vi "Dark Current Test_First_Half_Sub_VI.vi"(0 "VISA Refnum in":refnum<visa-resource-name>, 1 "Channel #":i32, 2 "dt (s)":i32, 3 "Barcodes in":string[](array[string]), 8 "N":i32) -> (10 "Actual Voltage Level (V)":dbl format="%#_13g", 12 "OVV?":bool=TRUE, 14 "Power Supply Trip":bool, 16 "OVC?":bool=TRUE, 17 "Boolean 2":bool, 18 "Actual Current Limit (nA)":dbl format="%#_13g", 19 "BoardHandle out 2":T1, 20 "VISA Refnum out":refnum<visa-resource-name>, 21 "Time Left (s)":dbl, 22 "Manual Measurments \nNeeded":bool, 23 "Barcodes out":string[](array[string]), 24 "Boolean":bool, 25 "Channel # 3":i32, 26 "Array":dbl[](array[numeric]), 27 "error out":errorcluster)   [LabVIEW 2018]
uses:
  Program Files (x86)/National Instruments/LabVIEW 2020/instr.lib/CAEN PSM/CAEN PSM.lvlib
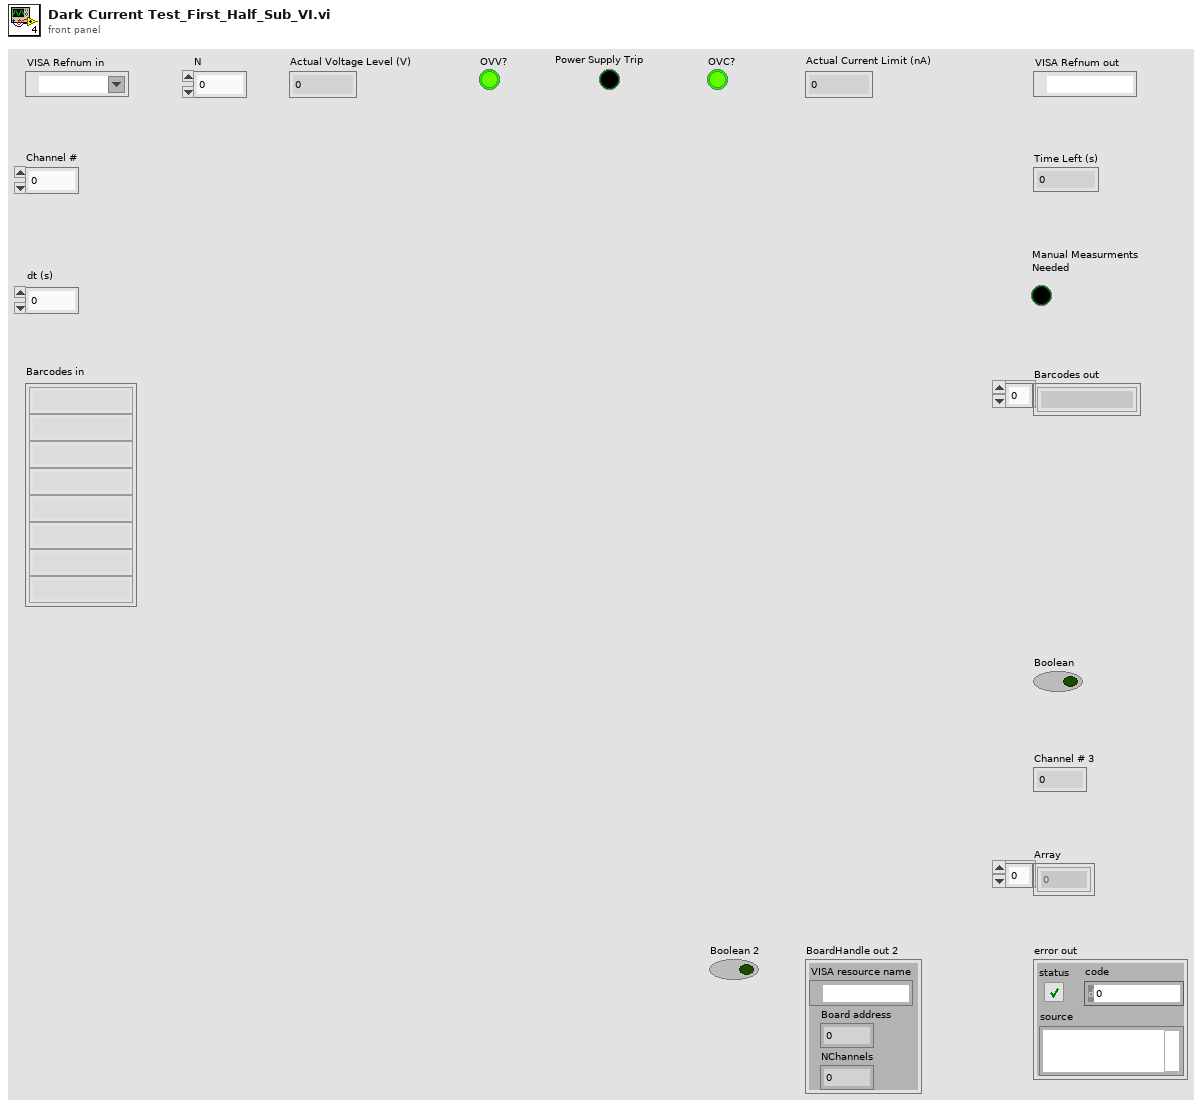
[diagram p1: front panel]
types:
  T1 = cluster{"VISA resource name":refnum<visa-resource-name>, "Board address":u8, "NChannels":u8}
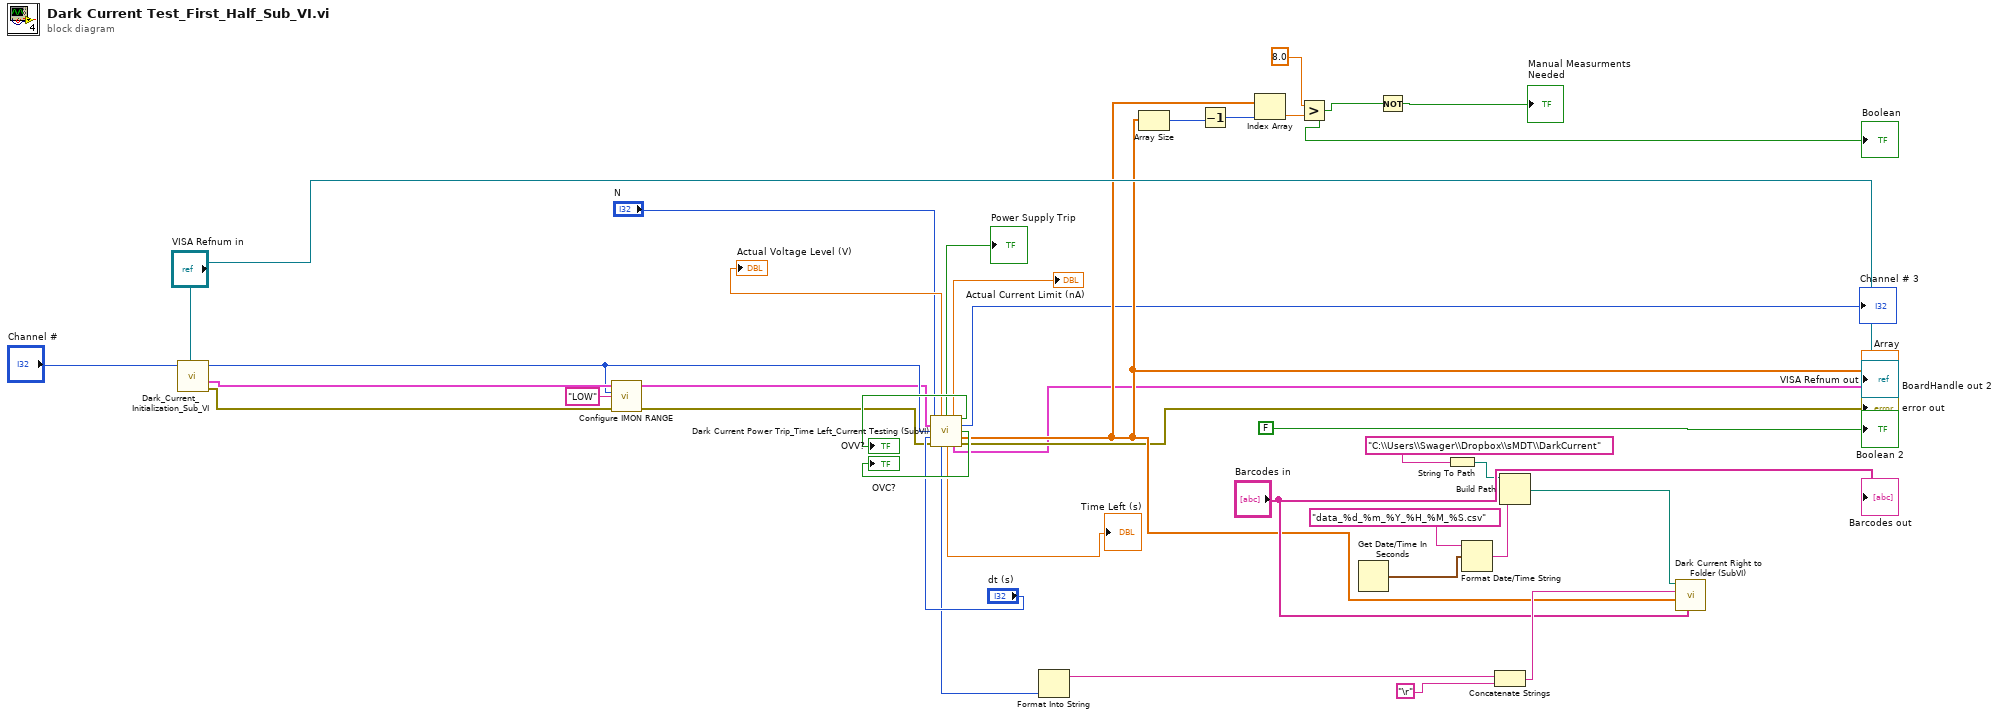
[diagram p0: block diagram]
diagram:
  n1 = call "Dark_Current_Initialization_Sub_VI.vi"("VISA resource name 2"="VISA Refnum in", "Channel #"="Channel #") -> ("error out"=w29:errorcluster, "BoardHandle out"=w28:T1, "Channel # 2"=w27:i32)  [unwired: 7 in]
  n2 = call "Configure IMON RANGE.vi"("error in (no error)"=w29, "IMon range (LOW)"="LOW", "Channel (0)"=w27, "BoardHandle"=w28) -> ("error out"=w8:errorcluster, "BoardHandle out"=w7:T1)  [unwired: 6 in]
  n3 = call "Dark Current Power Trip_Time Left_Current Testing (SubVI).vi"("N"="N", "BoardHandle in"=w7, "Channel # in"=w27, "dt (s) in"="dt (s)", "error in (no error)"=w8) -> ("Actual Voltage Level (V)"=→"Actual Voltage Level (V)":dbl, "Power Supply Trip"=→"Power Supply Trip":bool, "Actual Current Limit (nA)"=→"Actual Current Limit (nA)":dbl, "OVV?"=→"OVV?":bool, "Channel # 3"=→"Channel # 3":i32, "OVC?"=→"OVC?":bool, "Array"=w20:dbl[], "dt (s) out"=w21:i32, "Time Left (s)"=→"Time Left (s)":dbl, "BoardHandle out 2"=→"BoardHandle out 2":T1, "error out"=→"error out":errorcluster)
  "Array" <- w20
  n4 = Format Into String(w21) -> (resulting string=w25:string)  [unwired: 3 in, 1 out]
  n5 = Array Size(array=w20) -> (size(s)=w9:i32)
  n6 = Decrement(x=w9) -> (x-1=w10:i32)
  n7 = Index Array(array=w20, index=w10) -> (element=w11:dbl)
  n8 = Greater?(x=8.0, y=w11) -> (0:w12:bool)
  "Boolean" <- w12
  n9 = Get Date/Time In Seconds() -> (seconds since 1Jan1904=w17:timestamp)
  n10 = Not(x=w12) -> (.not. x?=→"Manual Measurments \nNeeded":bool)
  n11 = String To Path(string="C:\\Users\\Swager\\Dropbox\\sMDT\\DarkCurrent") -> (path=w18:path)
  n12 = Format Date/Time String(time format string (%c)="data_%d_%m_%Y_%H_%M_%S.csv", seconds (now)=w17) -> (date/time string=w16:string)  [unwired: 1 in]
  n13 = Concatenate Strings(w25, "\r") -> (w24:string)
  n14 = Build Path(base path=w18, name or relative path=w16) -> (appended path=w22:path)
  n15 = call "Dark Current Right to Folder (SubVI).vi"("Barcodes"="Barcodes in", "Array"=w20, "String"=w24, "appended path"=w22) -> ()  [unwired: 8 in]
  "VISA Refnum out" <- "VISA Refnum in"
  "Barcodes out" <- "Barcodes in"
  "Boolean 2" <- FALSE
